vi "op_biti_l2.vi"() -> ()   [LabVIEW 2009]
uses:
  <vilib>/Platform/portaccess.llb/Out Port8.vi
panel:
  in  "Knob":u8(knob)=3 scale=0.0..7.0
  out "Numeric":dbl=8.0
  out "Array":bool[](array[boolean])=[FALSE, FALSE, FALSE, FALSE, TRUE, FALSE, FALSE, FALSE]
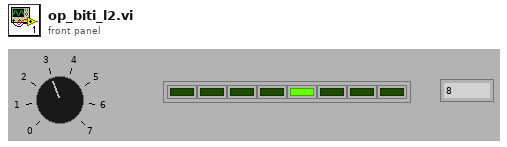
[diagram p1: front panel]
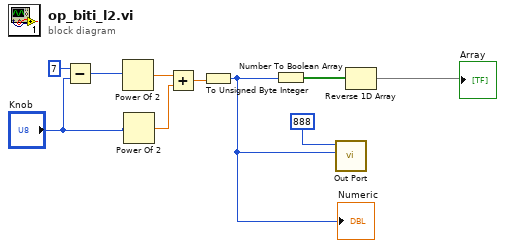
[diagram p0: block diagram]
diagram:
  n1 = Subtract(x=7, y="Knob") -> (x-y=w4:i32)
  n2 = Power Of 2(x=w4) -> (2^x=w3:dbl)
  n3 = Power Of 2(x="Knob") -> (2^x=w1:dbl)
  n4 = Add(x=w3, y=w1) -> (x+y=w2:dbl)
  n5 = To Unsigned Byte Integer(number=w2) -> (unsigned 8bit integer=w7:u8)
  "Numeric" <- w7
  n6 = Number To Boolean Array(number=w7) -> (Boolean array=w9:bool[])
  n7 = call-poly <vilib>:"Out Port.vi"("write value"=w7, "address"=888) -> ()  [unwired: 7 in, 1 out]
  n8 = Reverse 1D Array(array=w9) -> (reversed array=→"Array":bool[])
